vi "Create-buffer-action.vi"(8 "error in (no error)":errorcluster, 11 "Object ref in":T1) -> (0 "error out":errorcluster, 3 "Object ref out":T1)   [LabVIEW 2013, in "PowderDeposition.lvlib" / "PD-Main.lvclass"]
uses:
  PD-Main.lvclass
  Object-reference.ctl
  PD-Main.lvclass/PD-Main.ctl
  Motor/Motor.lvclass
  Action/Action.lvclass
  Assembly/Motor-assembly.lvclass
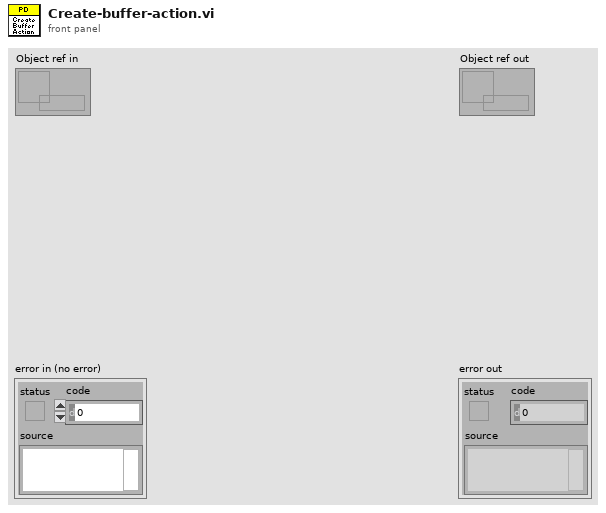
[diagram p1: front panel]
types:
  T1 = typedef "PowderDeposition.lvlib/PD-Main.lvclass/Object-reference.ctl" = refnum<data-value>
  T2 = typedef "PowderDeposition.lvlib/Action.lvclass/Motor-actions.ctl" = enum16{"Move - Absolute", "Move - Relative", "Move - Timer", "Wait", "Home", "Substrate", "Sieve", "Stop"}
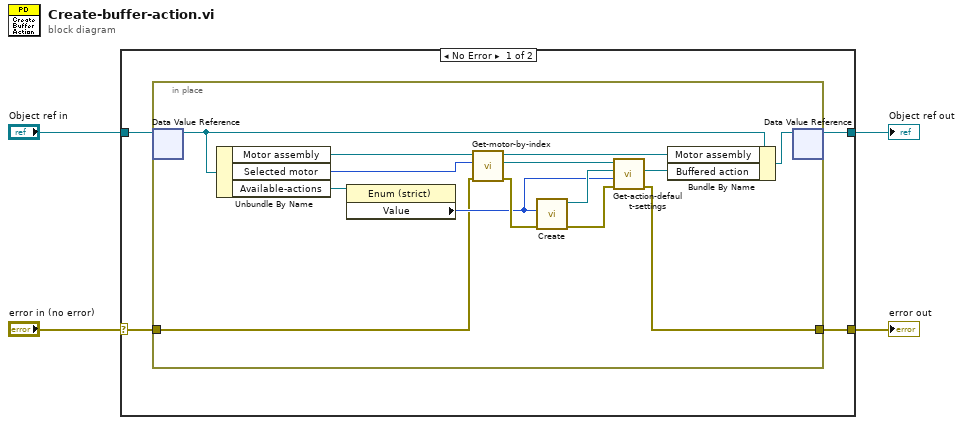
[diagram p0: block diagram]
diagram:
  n1 = case shown="No Error" "error in (no error)" {
    selector: "error in (no error)" -> [w8 w24]
    tunnel: [w7 w24] -> w3
    tunnel: [w5 w23] -> w1
    tunnel: "Object ref in" -> [w6 w23]
    frame No Error {
      n2 = in-place {
        in-place-border: w8 -> [w17]
        in-place-border: [w16] -> w7
        n3 = in-place-dvr #1(w6) -> (w12:refnum<class "PD-Main.lvclass">)  [unwired: 1 out]
        n4 = Unbundle By Name(w12) -> ("Motor assembly"=w15:refnum<class "Motor-assembly.lvclass">, "Selected motor"=w14:i32, "Available-actions"=w13:refnum<vi>)
        n5 = property class="Enum (strict)"(reference=w13) -> ("Value"=w18:T2)  [unwired: 1 in, 2 out]
        n6 = call "Get-motor-by-index.vi"("error in (no error)"=w17, "Index"=w14, "Available motors in"=w15) -> ("error out"=w20:errorcluster, "Motor"=w22:refnum<class "Motor.lvclass">, "Available motors out"=w11:refnum<class "Motor-assembly.lvclass">)  [unwired: 5 in, 1 out]
        n7 = call "Create.vi"("error in (no error)"=w20, "Action"=w18) -> ("error out"=w19:errorcluster, "Action out"=w21:refnum<class "Action.lvclass">)  [unwired: 8 in]
        n8 = call-dynamic "Get-action-default-settings.vi"("error in (no error)"=w19, "Motor actions"=w18, "Action in"=w21, "Motor in"=w22) -> ("error out"=w16:errorcluster, "Action"=w10:refnum<class "Action.lvclass">)  [unwired: 5 in, 1 out]
        n9 = Bundle By Name(cluster=w12, "Motor assembly"=w11, "Buffered action"=w10) -> (w9:refnum<class "PD-Main.lvclass">)
        n10 = in-place-dvr #1(w9) -> (w5:T1)  [unwired: 1 out]
      }
    }
    frame Error {
    }
  }
  "error out" <- w3
  "Object ref out" <- w1
